vi "arydh -- engine frontend.vi"   [LabVIEW 2019]
uses:
  publisher action.ctl
  nanocal/Nanocalorimetry/data/MCL.lvlibp/MCL library/MCL_DataRef.ctl
  nanocal/Nanocalorimetry/data/MCL.lvlibp
types:
  T1 = typedef "MCL.lvlibp/MCL_DataRef.ctl" = refnum<vi>
  T2 = typedef "publisher action.ctl" = enum16{"set", "get", "init", "check"}
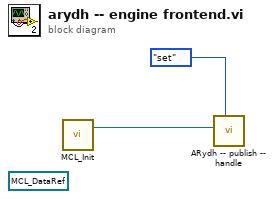
[diagram p0: block diagram]
diagram:
  (unwired) T1 refnum ("MCL object")
  n1 = call "MCL_Init.vi"() -> ("MCL object"=w1:T1)  [unwired: 2 in, 1 out]
  n2 = call "ARydh -- publish -- handle.vi"("publisher action"=publisher_action."set", "MCL object"=w1) -> ()  [unwired: 9 in, 1 out]
